vi "CowlStateController.vi"(0 "Desired State":string) -> (1 "Current State":string, 2 "Arrived":bool)   [LabVIEW 2019]
doc: "This VI manages the sequencing and transitions for the multi-position pneumatic cowl."
uses:
  outputs.vi
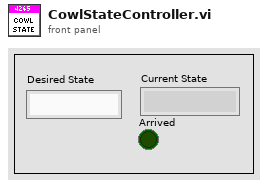
[diagram p1: front panel]
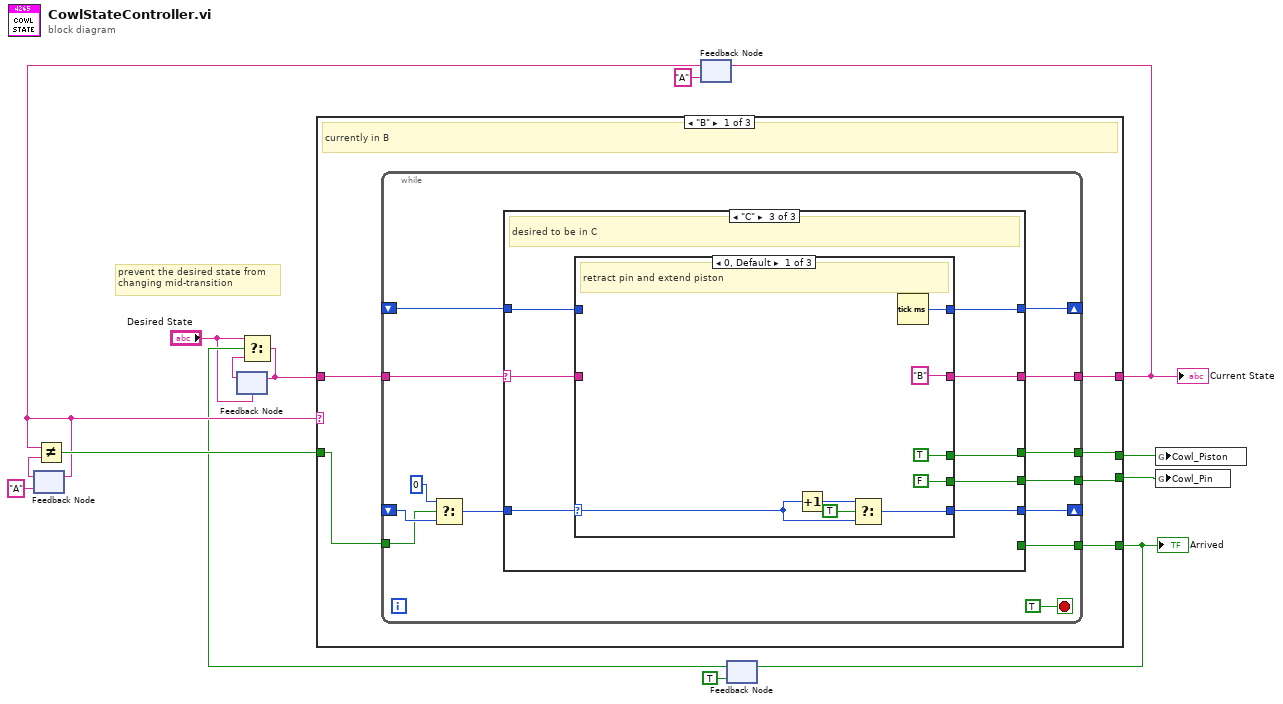
[diagram p0: block diagram]
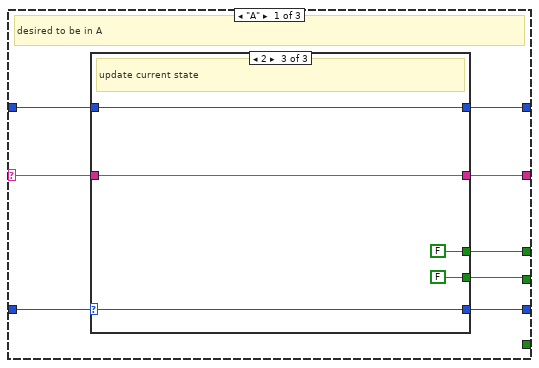
[diagram p2: hidden frame]
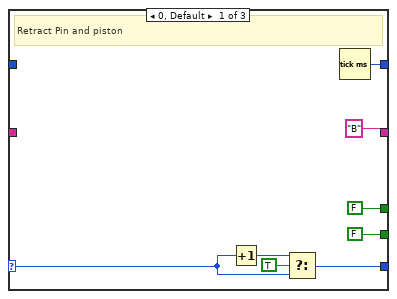
[diagram p3: hidden frame]
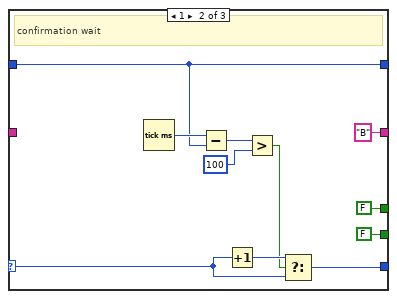
[diagram p4: hidden frame]
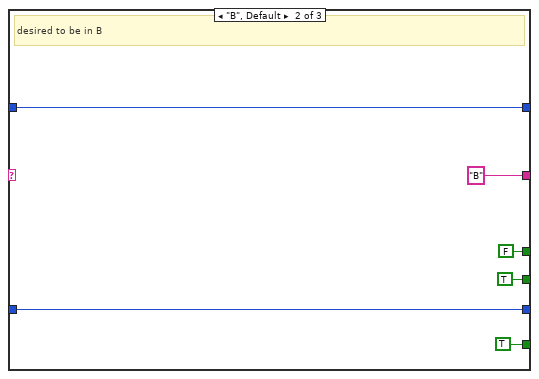
[diagram p5: hidden frame]
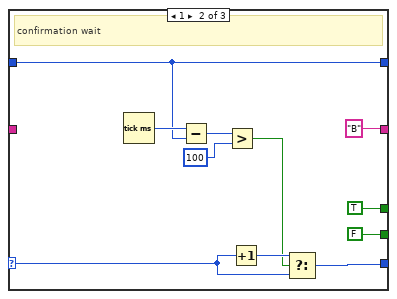
[diagram p6: hidden frame]
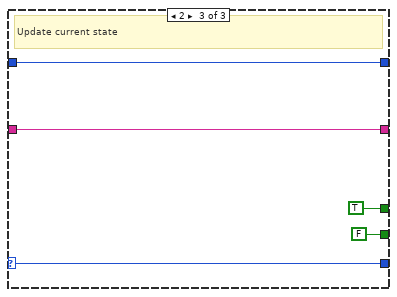
[diagram p7: hidden frame]
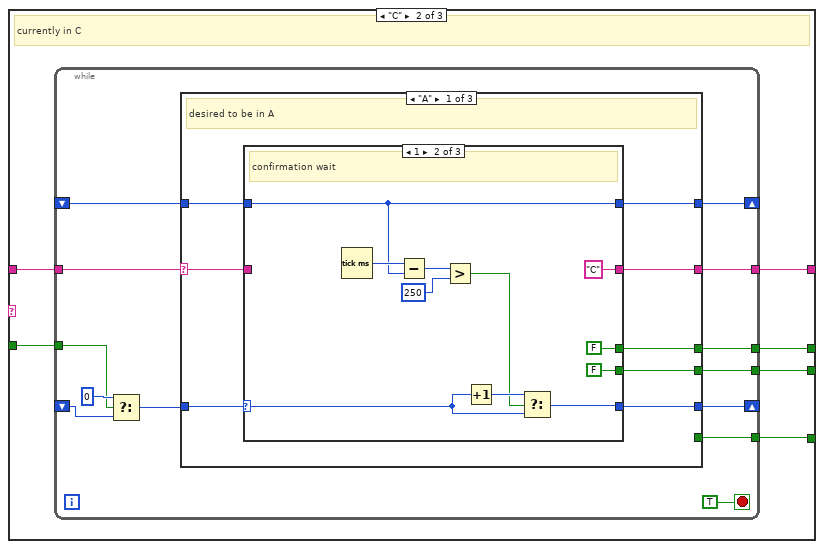
[diagram p8: hidden frame]
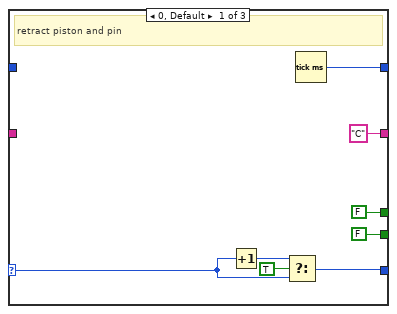
[diagram p9: hidden frame]
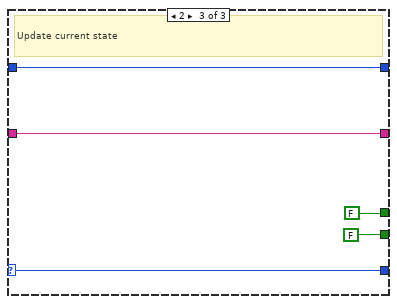
[diagram p10: hidden frame]
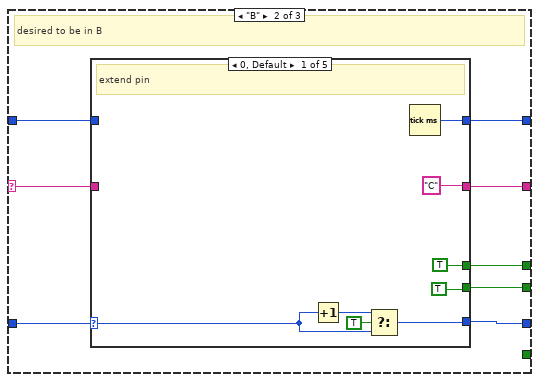
[diagram p11: hidden frame]
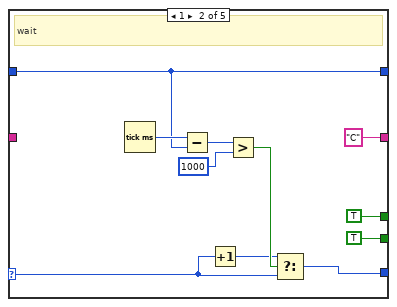
[diagram p12: hidden frame]
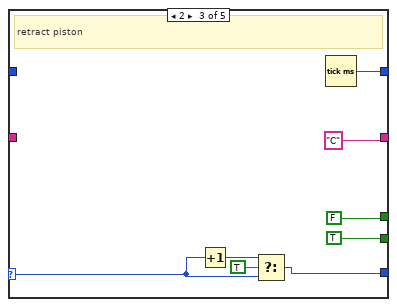
[diagram p13: hidden frame]
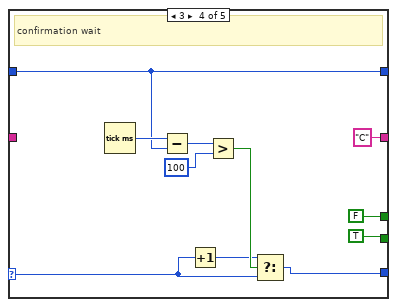
[diagram p14: hidden frame]
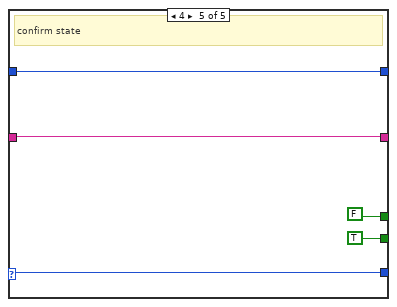
[diagram p15: hidden frame]
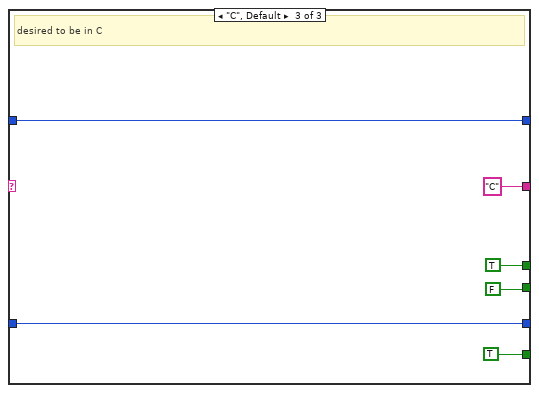
[diagram p16: hidden frame]
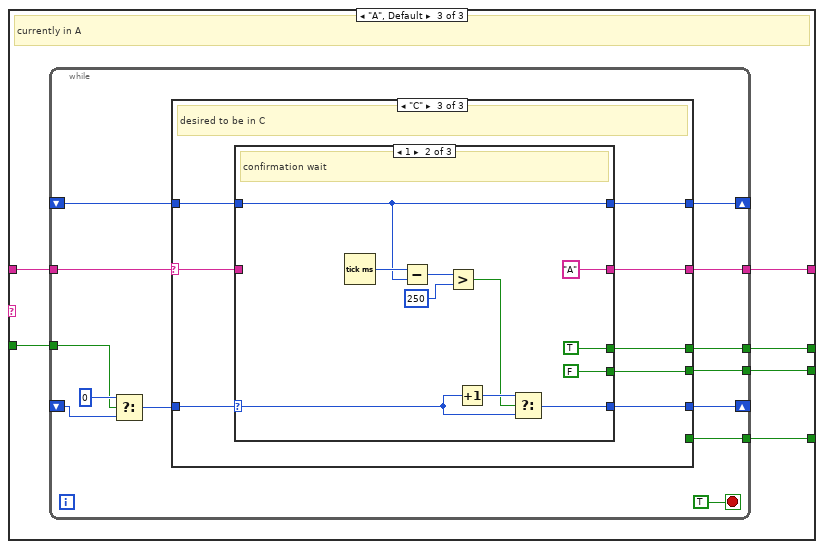
[diagram p17: hidden frame]
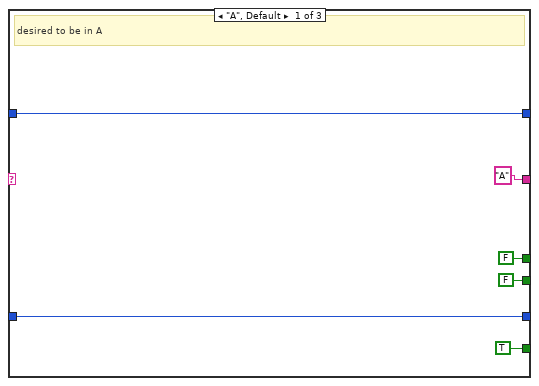
[diagram p18: hidden frame]
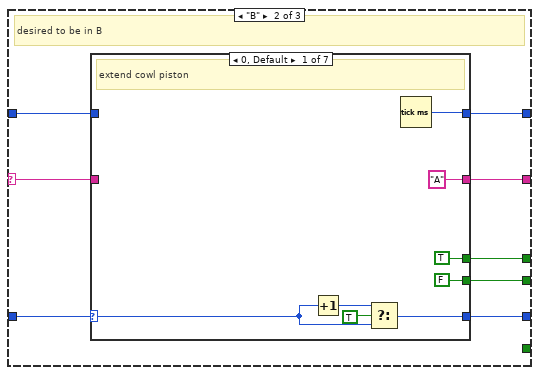
[diagram p19: hidden frame]
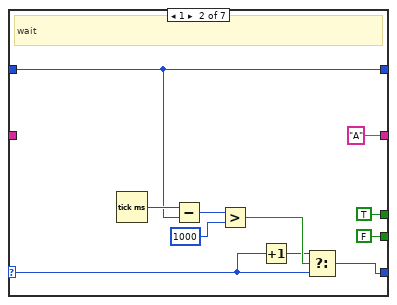
[diagram p20: hidden frame]
diagram:
  # "prevent the desired state from \nchanging mid-transition"
  n1 = feedback #1("A") -> (w12:string)
  n2 = feedback #2("Desired State") -> (w6:string)
  n3 = feedback #3("A") -> (w9:string)
  n4 = feedback-in #1(w9) -> ()
  n5 = Not Equal?(x=w9, y=w12) -> (x != y?=w11:bool)
  n6 = feedback #4(TRUE) -> (w7:bool)
  n7 = Select(t="Desired State", s=w7, f=w6) -> (s? t:f=w4:string)
  n8 = feedback-in #2(w4) -> ()
  n9 = case shown="\"B\"" w9 {
    tunnel: [w18 w108 w217] -> w13
    tunnel: [w19 w109 w215] -> w10
    tunnel: [w20 w107 w216] -> w14
    tunnel: w11 -> [w17 w106 w214]
    tunnel: w4 -> [w16 w105 w213]
    tunnel: [w15 w104 w212] -> w8
    frame "B" {
      # "currently in B"
      n10 = while {
        shift-right: [w30] -> _
        shift-left: _ -> [w32]
        tunnel: [w28] -> w18
        tunnel: [w27] -> w19
        tunnel: [w26] -> w20
        tunnel: w17 -> [w25]
        tunnel: w16 -> [w24]
        tunnel: [w23] -> w15
        shift-right: [w22] -> _
        shift-left: _ -> [w21]
        stop <- TRUE stop-if-true
        n11 = Select(t=0, s=w25, f=w32) -> (s? t:f=w31:i32)
        n12 = case shown="\"C\"" w24 {
          selector: w24 -> [w36 _ w74]
          tunnel: w31 -> [w40 w71 w75]
          tunnel: [w41 w71 w76] -> w30
          tunnel: [w39 FALSE w78] -> w28
          tunnel: [w38 "B" w79] -> w27
          tunnel: [w37 TRUE w77] -> w26
          tunnel: [_ TRUE _] -> w23
          tunnel: [w35 w66 w73] -> w22
          tunnel: w21 -> [w34 w66 w72]
          frame "A" {
            # "desired to be in A"
            n13 = case shown="2" w40 {
              selector: w40 -> [w49 w54 w65]
              tunnel: [w48 w53 w65] -> w41
              tunnel: [FALSE FALSE FALSE] -> w39
              tunnel: ["B" "B" w62] -> w38
              tunnel: [FALSE FALSE FALSE] -> w37
              tunnel: w36 -> [_ _ w62]
              tunnel: [w42 w57 w61] -> w35
              tunnel: w34 -> [_ w57 w61]
              frame 0, Default {
                # "Retract Pin and piston"
                n14 = Increment(x=w49) -> (x+1=w47:i32)
                n15 = Select(t=w47, s=TRUE, f=w49) -> (s? t:f=w48:i32)
                n16 = Tick Count (ms)() -> (millisecond timer value=w42:u32)
              }
              frame 1 {
                # "confirmation wait"
                n17 = Tick Count (ms)() -> (millisecond timer value=w59:u32)
                n18 = Subtract(x=w59, y=w57) -> (x-y=w60:u32)
                n19 = Increment(x=w54) -> (x+1=w55:i32)
                n20 = Greater?(x=w60, y=u32 100) -> (0:w52:bool)
                n21 = Select(t=w55, s=w52, f=w54) -> (s? t:f=w53:i32)
              }
              frame 2 {
                # "update current state"
              }
            }
          }
          frame "B", Default {
            # "desired to be in B"
          }
          frame "C" {
            # "desired to be in C"
            n22 = case shown="0, Default" w75 {
              selector: w75 -> [w87 w98 w103]
              tunnel: [w86 w97 w103] -> w76
              tunnel: [TRUE TRUE TRUE] -> w78
              tunnel: ["B" "B" w99] -> w79
              tunnel: [FALSE FALSE FALSE] -> w77
              tunnel: w74 -> [_ _ w99]
              tunnel: [w80 w89 w100] -> w73
              tunnel: w72 -> [_ w89 w100]
              frame 0, Default {
                # "retract pin and extend piston"
                n23 = Increment(x=w87) -> (x+1=w85:i32)
                n24 = Select(t=w85, s=TRUE, f=w87) -> (s? t:f=w86:i32)
                n25 = Tick Count (ms)() -> (millisecond timer value=w80:u32)
              }
              frame 1 {
                # "confirmation wait"
                n26 = Tick Count (ms)() -> (millisecond timer value=w91:u32)
                n27 = Subtract(x=w91, y=w89) -> (x-y=w92:u32)
                n28 = Greater?(x=w92, y=u32 100) -> (0:w88:bool)
                n29 = Increment(x=w98) -> (x+1=w96:i32)
                n30 = Select(t=w96, s=w88, f=w98) -> (s? t:f=w97:i32)
              }
              frame 2 {
                # "Update current state"
              }
            }
          }
        }
      }
    }
    frame "C" {
      # "currently in C"
      n31 = while {
        shift-right: [w121] -> _
        shift-left: _ -> [w122]
        shift-right: [w117] -> _
        shift-left: _ -> [w119]
        tunnel: [w115] -> w108
        tunnel: [w114] -> w109
        tunnel: [w113] -> w107
        tunnel: w106 -> [w112]
        tunnel: w105 -> [w111]
        tunnel: [w110] -> w104
        stop <- TRUE stop-if-true
        n32 = Select(t=0, s=w112, f=w119) -> (s? t:f=w118:i32)
        n33 = case shown="\"A\"" w111 {
          selector: w111 -> [w123 w155 _]
          tunnel: w122 -> [w125 w159 w211]
          tunnel: [w128 w158 w211] -> w121
          tunnel: w118 -> [w130 w161 w210]
          tunnel: [w129 w162 w210] -> w117
          tunnel: [w127 w160 TRUE] -> w115
          tunnel: [w126 w157 "C"] -> w114
          tunnel: [w124 w156 FALSE] -> w113
          tunnel: [_ _ TRUE] -> w110
          frame "A" {
            # "desired to be in A"
            n34 = case shown="1" w130 {
              selector: w130 -> [w138 w149 w154]
              tunnel: [w137 w148 w154] -> w129
              tunnel: [FALSE FALSE FALSE] -> w127
              tunnel: [w133 w140 w153] -> w128
              tunnel: ["C" "C" w150] -> w126
              tunnel: w125 -> [_ w140 w153]
              tunnel: [FALSE FALSE FALSE] -> w124
              tunnel: w123 -> [_ _ w150]
              frame 0, Default {
                # "retract piston and pin"
                n35 = Increment(x=w138) -> (x+1=w136:i32)
                n36 = Select(t=w136, s=TRUE, f=w138) -> (s? t:f=w137:i32)
                n37 = Tick Count (ms)() -> (millisecond timer value=w133:u32)
              }
              frame 1 {
                # "confirmation wait"
                n38 = Tick Count (ms)() -> (millisecond timer value=w142:u32)
                n39 = Subtract(x=w142, y=w140) -> (x-y=w143:u32)
                n40 = Greater?(x=w143, y=u32 250) -> (0:w139:bool)
                n41 = Increment(x=w149) -> (x+1=w147:i32)
                n42 = Select(t=w147, s=w139, f=w149) -> (s? t:f=w148:i32)
              }
              frame 2 {
                # "Update current state"
              }
            }
          }
          frame "B" {
            # "desired to be in B"
            n43 = case shown="0, Default" w161 {
              selector: w161 -> [w170 w176 w186 w194 w202]
              tunnel: [w169 w175 w185 w193 w202] -> w162
              tunnel: [TRUE TRUE FALSE FALSE FALSE] -> w160
              tunnel: w159 -> [_ w179 _ w195 w205]
              tunnel: [w163 w179 w182 w195 w205] -> w158
              tunnel: ["C" "C" "C" "C" w201] -> w157
              tunnel: [TRUE TRUE TRUE TRUE TRUE] -> w156
              tunnel: w155 -> [_ _ _ _ w201]
              frame 0, Default {
                # "extend pin"
                n44 = Increment(x=w170) -> (x+1=w168:i32)
                n45 = Select(t=w168, s=TRUE, f=w170) -> (s? t:f=w169:i32)
                n46 = Tick Count (ms)() -> (millisecond timer value=w163:u32)
              }
              frame 1 {
                # "wait"
                n47 = Tick Count (ms)() -> (millisecond timer value=w181:u32)
                n48 = Subtract(x=w181, y=w179) -> (x-y=w180:u32)
                n49 = Increment(x=w176) -> (x+1=w174:i32)
                n50 = Greater?(x=w180, y=u32 1000) -> (0:w178:bool)
                n51 = Select(t=w174, s=w178, f=w176) -> (s? t:f=w175:i32)
              }
              frame 2 {
                # "retract piston"
                n52 = Increment(x=w186) -> (x+1=w188:i32)
                n53 = Select(t=w188, s=TRUE, f=w186) -> (s? t:f=w185:i32)
                n54 = Tick Count (ms)() -> (millisecond timer value=w182:u32)
              }
              frame 3 {
                # "confirmation wait"
                n55 = Tick Count (ms)() -> (millisecond timer value=w200:u32)
                n56 = Subtract(x=w200, y=w195) -> (x-y=w199:u32)
                n57 = Increment(x=w194) -> (x+1=w196:i32)
                n58 = Greater?(x=w199, y=u32 100) -> (0:w198:bool)
                n59 = Select(t=w196, s=w198, f=w194) -> (s? t:f=w193:i32)
              }
              frame 4 {
                # "confirm state"
              }
            }
          }
          frame "C", Default {
            # "desired to be in C"
          }
        }
      }
    }
    frame "A", Default {
      # "currently in A"
      n60 = while {
        shift-right: [w229] -> _
        shift-left: _ -> [w230]
        shift-right: [w225] -> _
        shift-left: _ -> [w227]
        tunnel: [w223] -> w217
        tunnel: [w222] -> w215
        tunnel: [w221] -> w216
        tunnel: w214 -> [w220]
        tunnel: w213 -> [w219]
        tunnel: [w218] -> w212
        stop <- TRUE stop-if-true
        n61 = Select(t=0, s=w220, f=w227) -> (s? t:f=w226:i32)
        n62 = case shown="\"C\"" w219 {
          selector: w219 -> [_ w237 w307]
          tunnel: w230 -> [w236 w241 w309]
          tunnel: [w236 w240 w312] -> w229
          tunnel: w226 -> [w235 w243 w314]
          tunnel: [w235 w244 w313] -> w225
          tunnel: [FALSE w242 w311] -> w223
          tunnel: ["A" w239 w310] -> w222
          tunnel: [FALSE w238 w308] -> w221
          tunnel: [TRUE _ _] -> w218
          frame "A", Default {
            # "desired to be in A"
          }
          frame "B" {
            # "desired to be in B"
            n63 = case shown="0, Default" w243 {
              selector: w243 -> [w252 w258 w268 w276 w286 w298 w306]
              tunnel: [w251 w257 w267 w275 w287 w299 w306] -> w244
              tunnel: [TRUE TRUE TRUE TRUE FALSE FALSE FALSE] -> w242
              tunnel: w241 -> [_ w261 _ w277 _ w292 w305]
              tunnel: [w245 w261 w264 w277 w283 w292 w305] -> w240
              tunnel: ["A" "A" "A" "A" "A" "A" w302] -> w239
              tunnel: [FALSE FALSE TRUE TRUE TRUE TRUE TRUE] -> w238
              tunnel: w237 -> [_ _ _ _ _ _ w302]
              frame 0, Default {
                # "extend cowl piston"
                n64 = Increment(x=w252) -> (x+1=w250:i32)
                n65 = Select(t=w250, s=TRUE, f=w252) -> (s? t:f=w251:i32)
                n66 = Tick Count (ms)() -> (millisecond timer value=w245:u32)
              }
              frame 1 {
                # "wait"
                n67 = Tick Count (ms)() -> (millisecond timer value=w263:u32)
                n68 = Subtract(x=w263, y=w261) -> (x-y=w262:u32)
                n69 = Greater?(x=w262, y=u32 1000) -> (0:w260:bool)
                n70 = Increment(x=w258) -> (x+1=w256:i32)
                n71 = Select(t=w256, s=w260, f=w258) -> (s? t:f=w257:i32)
              }
              frame 2 {
                # "extend cowl pin"
                n72 = Increment(x=w268) -> (x+1=w270:i32)
                n73 = Select(t=w270, s=TRUE, f=w268) -> (s? t:f=w267:i32)
                n74 = Tick Count (ms)() -> (millisecond timer value=w264:u32)
              }
              frame 3 {
                # "wait"
                n75 = Tick Count (ms)() -> (millisecond timer value=w282:u32)
                n76 = Subtract(x=w282, y=w277) -> (x-y=w281:u32)
                n77 = Increment(x=w276) -> (x+1=w278:i32)
                n78 = Greater?(x=w281, y=u32 1000) -> (0:w280:bool)
                n79 = Select(t=w278, s=w280, f=w276) -> (s? t:f=w275:i32)
              }
              frame 4 {
                # "retract cowl piston"
                n80 = Increment(x=w286) -> (x+1=w289:i32)
                n81 = Select(t=w289, s=TRUE, f=w286) -> (s? t:f=w287:i32)
                n82 = Tick Count (ms)() -> (millisecond timer value=w283:u32)
              }
              frame 5 {
                # "confirmation wait"
                n83 = Tick Count (ms)() -> (millisecond timer value=w295:u32)
                n84 = Subtract(x=w295, y=w292) -> (x-y=w294:u32)
                n85 = Greater?(x=w294, y=u32 100) -> (0:w291:bool)
                n86 = Increment(x=w298) -> (x+1=w300:i32)
                n87 = Select(t=w300, s=w291, f=w298) -> (s? t:f=w299:i32)
              }
              frame 6 {
                # "Update current state"
              }
            }
          }
          frame "C" {
            # "desired to be in C"
            n88 = case shown="1" w314 {
              selector: w314 -> [w322 w333 w338]
              tunnel: [w321 w332 w338] -> w313
              tunnel: [TRUE TRUE TRUE] -> w311
              tunnel: [w317 w324 w337] -> w312
              tunnel: ["A" "A" w334] -> w310
              tunnel: w309 -> [_ w324 w337]
              tunnel: [FALSE FALSE FALSE] -> w308
              tunnel: w307 -> [_ _ w334]
              frame 0, Default {
                # "extend cowl piston"
                n89 = Increment(x=w322) -> (x+1=w320:i32)
                n90 = Select(t=w320, s=TRUE, f=w322) -> (s? t:f=w321:i32)
                n91 = Tick Count (ms)() -> (millisecond timer value=w317:u32)
              }
              frame 1 {
                # "confirmation wait"
                n92 = Tick Count (ms)() -> (millisecond timer value=w327:u32)
                n93 = Subtract(x=w327, y=w324) -> (x-y=w326:u32)
                n94 = Greater?(x=w326, y=u32 250) -> (0:w323:bool)
                n95 = Increment(x=w333) -> (x+1=w331:i32)
                n96 = Select(t=w331, s=w323, f=w333) -> (s? t:f=w332:i32)
              }
              frame 2 {
                # "Update current state"
              }
            }
          }
        }
      }
    }
  }
  "Current State" <- w10
  "Arrived" <- w8
  n97 = feedback-in #3(w10) -> ()
  n98 = feedback-in #4(w8) -> ()
  n99 = global write "outputs.vi" "Cowl_Piston"(w13) -> ()
  n100 = global write "outputs.vi" "Cowl_Pin"(w14) -> ()
